vi "Analysis for plotting.vi"() -> (1 "Index of Hist and Spec":i32[](array[numeric]))   [LabVIEW 2022 SP3]
uses:
  Controls/Graph_Type.ctl
  Globals/Meas_global.vi
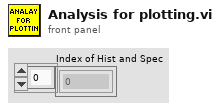
[diagram p1: front panel]
types:
  T1 = typedef "Graph_Type.ctl" = enum16{"Show no graph", "Voltage trace", "Velocity trace", "Vel histogram", "Spectrum", "f.E(f) v Log f", "Auto-Corr"}
  T2 = cluster{"Plot 1":u16, "Plot 2":u16, "Save graph":u16, "Plot Type":T1}
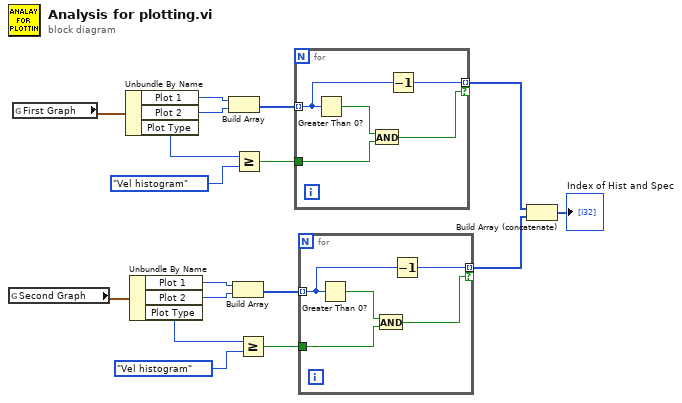
[diagram p0: block diagram]
diagram:
  n1 = global read "Meas_global.vi" "Second Graph"() -> (w4:T2)
  n2 = global read "Meas_global.vi" "First Graph"() -> (w17:T2)
  n3 = Unbundle By Name(w17) -> ("Plot 1"=w14:u16, "Plot 2"=w13:u16, "Plot Type"=w16:T1)
  n4 = Unbundle By Name(w4) -> ("Plot 1"=w7:u16, "Plot 2"=w8:u16, "Plot Type"=w5:T1)
  n5 = Build Array(w14, w13) -> (w12:u16[])
  n6 = Build Array(w7, w8) -> (w9:u16[])
  n7 = Greater Or Equal?(x=w16, y=Graph_Type."Vel histogram" ("Plot Type")) -> (x >= y?=w11:bool)
  n8 = Greater Or Equal?(x=w5, y=Graph_Type."Vel histogram" ("Plot Type")) -> (x >= y?=w10:bool)
  n9 = for {
    tunnel: w12 -> [w20] mode=indexing
    tunnel: w11 -> [w21]
    tunnel: [w19] -> w3 mode=indexing if=w18
    n10 = Greater Than 0?(x=w20) -> (x > 0?=w22:bool)
    n11 = And(x=w22, y=w21) -> (x .and. y?=w18:bool)
    n12 = Decrement(x=w20) -> (x-1=w19:u16)
  }
  n13 = for {
    tunnel: w9 -> [w25] mode=indexing
    tunnel: w10 -> [w26]
    tunnel: [w24] -> w2 mode=indexing if=w23
    n14 = Greater Than 0?(x=w25) -> (x > 0?=w27:bool)
    n15 = And(x=w27, y=w26) -> (x .and. y?=w23:bool)
    n16 = Decrement(x=w25) -> (x-1=w24:u16)
  }
  n17 = Build Array (concatenate)(w3, w2) -> (→"Index of Hist and Spec":u16[])
